vi "SPC_read_fifo_to_stream.vi"(6 "Stream Handle":i16, 7 "MaxCount":u32, 8 "Error In":errorcluster, 10 "Module No":i16, 11 "DLL Path":path) -> (0 "Error Out":errorcluster, 2 "Module No":i16, 3 "DLL Path":path, 4 "Stream Handle":i16, 5 "Count":u32)   [LabVIEW 2023]
doc: "The procedure can be used to add events data to the opened ‘buffered’ photons stream defined by handle ‘stream_hndl’. Photons are read from the FIFO on SPC module ‘mod_no’ during running FIFO measurement.\n\nMaxCount is the max expected number of events to transfer; used for buffer allocation.\nThe ‘Count’ variable is filled on exit with the number of 16-bit words added to the stream. See also the description of SPC_read_fifo procedure because it is called internally. Photons data read from FIFO are added to DLL internal buffers which have size between STREAM_MIN_BUF_SIZE and STREAM_MAX_BUF_SIZE. Internal buffers are allocated by DLL when required.\n\nMaximum size of allocated stream buffers is equal STREAM_MAX_SIZE32 for 32-bit DLL and STREAM_MAX_SIZE64 for 64-bit DLL. The buffers are freed, when the stream is closed (SPCM_close_phot_stream) or when, during SPC_get_photons_from_stream call, all photons from the current buffer are extracted ( if an option FREE_BUF_STREAM ( bit 13 in ‘stream_type’ ) is set).\n\nProcedure returns error, if ‘stream_hndl’ is not the handle of the stream opened using SPC_init_buf_stream function.\n\ninfo@becker-hickl.com"
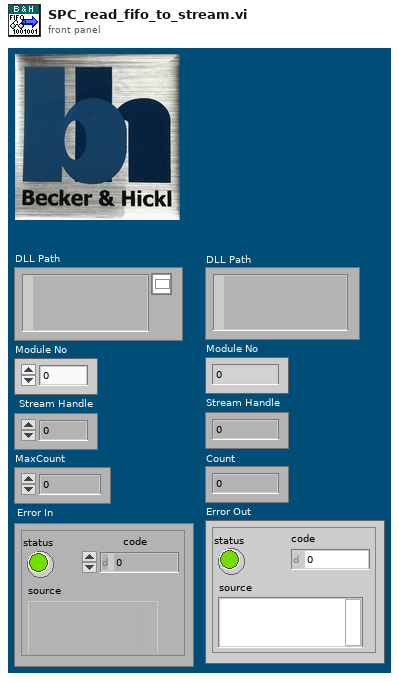
[diagram p1: front panel]
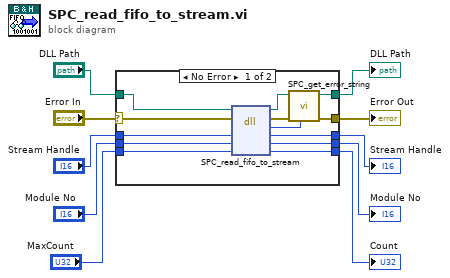
[diagram p0: block diagram]
diagram:
  n1 = case shown="No Error" "Error In" {
    selector: "Error In" -> [w23 w28]
    tunnel: [w21 w28] -> w9
    tunnel: "DLL Path" -> [w20 w27]
    tunnel: [w18 w27] -> w7
    tunnel: "Module No" -> [w17 w25]
    tunnel: "Stream Handle" -> [w16 w24]
    tunnel: [w15 w26] -> w4
    tunnel: "MaxCount" -> [w14 w26]
    tunnel: [w13 w25] -> w2
    tunnel: [w11 w24] -> w1
    frame No Error {
      n2 = dll-call lib="D:/spcm/lib/lab_view/lv10.0/spcm32.dll" fn="SPC_read_fifo_to_stream"(path in=w20, error in=w23, "stream_hndl"=w16, "mod_no"=w17, "count"=w14) -> (path out=w19:path, error out=w22:errorcluster, "return type"=w12:i16, "stream_hndl"=w11:i16, "mod_no"=w13:i16, "count"=w15:u32)  [unwired: 1 in]
      n3 = call "SPC_get_error_string.vi"("ErrorID"=w12, "Error In"=w22, "DLL Path"=w19) -> ("Error Out"=w21:errorcluster, "DLL Path"=w18:path)  [unwired: 6 in, 1 out]
    }
    frame Error {
    }
  }
  "DLL Path" <- w7
  "Error Out" <- w9
  "Count" <- w4
  "Module No" <- w2
  "Stream Handle" <- w1
